vi "Winch_RT.vi"() -> ()   [LabVIEW 2018]
uses:
  Custom Controls/Address_Value Command Cluster.ctl
  Custom Controls/Counter.ctl
  Custom Controls/Slave_ID.ctl
  Custom Controls/MotorStatusCluster.ctl
  <vilib>/Platform/TimedLoop/XDataNode/timing_clust.ctl
  <vilib>/Platform/TimedLoop/XDataNode/nitl_modes.ctl
  <vilib>/Platform/TimedLoop/XDataNode/wakeup.ctl
  <vilib>/myRIO/Common/Instrument Driver Framework/myRIO v1.0/Encoder/typedefs/Encoder Signal Mode.ctl
  <vilib>/myRIO/Instrument Drivers/Onboard IO/Encoder/typedefs/Encoder Reference.ctl
  <vilib>/myRIO/Common/Instrument Driver Framework/Utilities/typedefs/myRIO Generic Hardware Reference.ctl
  <vilib>/myRIO/Common/Instrument Driver Framework/Utilities/typedefs/Hardware Version Enum.ctl
  <vilib>/myRIO/Common/Instrument Driver Framework/Utilities/typedefs/myRIO v1.0 Reference.ctl
  <vilib>/myRIO/Common/Instrument Driver Framework/Utilities/typedefs/Generic FPGA Reference.ctl
  <vilib>/myRIO/Common/Instrument Driver Framework/myRIO v1.0/Encoder/typedefs/Encoder Channels Enum.ctl
  <vilib>/myRIO/Common/Instrument Driver Framework/myRIO v1.0/Encoder/typedefs/Encoder Configuration v1.0.ctl
  <vilib>/userdefined/High Color/nirio_resource_hc.ctl
  <vilib>/myRIO/Instrument Drivers/Onboard IO/DIO/typedefs/DIO Reference.ctl
  <vilib>/myRIO/Common/Instrument Driver Framework/myRIO v1.0/DIO/typedefs/DIO Channels List.ctl
  <vilib>/myRIO/Common/Instrument Driver Framework/myRIO v1.0/DIO/typedefs/DIO Channels Enum.ctl
  <vilib>/myRIO/Common/Instrument Driver Framework/Utilities/vis/Is FPGA Ref Available.vi
  <vilib>/myRIO/Common/Instrument Driver Framework/myRIO v1.0/Encoder/vis/myRIO v1.1 Open Encoder.vi
  <vilib>/myRIO/Instrument Drivers/Onboard IO/Encoder/vis/Read.vi
  <vilib>/myRIO/Common/Instrument Driver Framework/myRIO v1.0/DIO/vis/myRIO v1.1 Open DIO.vi
  <vilib>/myRIO/Instrument Drivers/Onboard IO/DIO/vis/Read.vi
  <vilib>/myRIO/Common/Instrument Driver Framework/Utilities/vis/Validate Channels.vi
  <vilib>/myRIO/Common/Instrument Driver Framework/myRIO v1.0/Encoder/vis/myRIO v1.0 Reserve Encoder.vi
  <vilib>/myRIO/Common/Instrument Driver Framework/myRIO v1.0/DIO/vis/myRIO v1.0 Reserve DIO.vi
  <vilib>/myRIO/Common/Instrument Driver Framework/myRIO v1.0/UART/vis/myRIO v1.0 Close UART.vi
  <vilib>/myRIO/Common/Instrument Driver Framework/myRIO v1.0/Encoder/vis/myRIO v1.0 Build MUX Configuration Encoder.vi
  <vilib>/myRIO/Common/Instrument Driver Framework/myRIO v1.0/Resource Manager/vis/myRIO v1.0 Reserve Channel List.vi
  <vilib>/myRIO/Common/Instrument Driver Framework/myRIO v1.0/DIO/vis/myRIO v1.0 Build MUX Configuration DIO.vi
  <vilib>/myRIO/Common/Instrument Driver Framework/myRIO v1.0/Resource Manager/vis/myRIO v1.0 Create Configuration List.vi
  <vilib>/myRIO/Common/Instrument Driver Framework/myRIO v1.0/Resource Manager/vis/myRIO v1.0 Reserve Channel.vi
  <vilib>/myRIO/Common/Instrument Driver Framework/myRIO v1.0/Resource Manager/vis/myRIO v1.0 Unreserve Channel.vi
  <vilib>/myRIO/Common/Instrument Driver Framework/myRIO v1.0/Resource Manager/vis/myRIO v1.0 Build Mutex Name.vi
  <vilib>/Plasmionique/MB Master/MB_Master_Serial/MB_Master_Serial.lvclass
  D:/Program Files (x86)/National Instruments/LabVIEW 2018/vi.lib/Plasmionique/MB Master/MB_Master/MB_Master.lvclass
  <vilib>/Utility/VariantDataType/GetNumericInfo.vi
  <vilib>/Utility/error.llb/Error Cluster From Error Code.vi
  <vilib>/myRIO/Common/Instrument Driver Framework/myRIO v1.0/myRIO v1.1 Open.vi
  <vilib>/myRIO/Common/Instrument Driver Framework/Utilities/vis/IO Manager.vi
  <vilib>/myRIO/Common/Instrument Driver Framework/Utilities/vis/Configuration Manager.vi
  <vilib>/myRIO/Common/Instrument Driver Framework/myRIO v1.0/Resource Manager/vis/myRIO v1.0 Configure IO.vi
  <vilib>/myRIO/Common/Instrument Driver Framework/myRIO v1.0/myRIO v1.0 Close.vi
  <vilib>/myRIO/Common/Instrument Driver Framework/myRIO v1.0/Encoder/vis/myRIO v1.0 Configure Encoder.vi
  <vilib>/myRIO/Common/Instrument Driver Framework/myRIO v1.0/Encoder/vis/myRIO v1.0 Read Encoder.vi
  <vilib>/myRIO/Common/Instrument Driver Framework/myRIO v1.0/DIO/vis/myRIO v1.0 Read DIO.vi
  <vilib>/myRIO/Common/Instrument Driver Framework/Utilities/vis/FPGA Ref Manager.vi
  <vilib>/myRIO/Common/Instrument Driver Framework/myRIO v1.0/myRIO v1.0 Reset FPGA.vi
  <vilib>/myRIO/Common/Instrument Driver Framework/myRIO v1.0/IRQ/vis/myRIO v1.0 IRQ Info FGV.vi
  <vilib>/myRIO/Common/Instrument Driver Framework/myRIO v1.0/IRQ/vis/myRIO v1.0 Timer IRQ Info FGV.vi
  <vilib>/myRIO/Common/Instrument Driver Framework/myRIO v1.0/IRQ/vis/myRIO v1.0 ISR Agent.vi
  <vilib>/platform/TimedLoop/XDataNode/XDataNode.xnode
  <vilib>/myRIO/Express VI/Onboard IO/Encoder/Encoder Express VI.xnode
  <vilib>/myRIO/Instrument Drivers/Onboard IO/Encoder/vis/myRIO Encoder Open.xnode
  <vilib>/myRIO/Express VI/Onboard IO/DI/DI Express VI.xnode
  <vilib>/myRIO/Instrument Drivers/Onboard IO/DIO/vis/myRIO DIO Open.xnode
  <vilib>/Plasmionique/MB Master/MB Master.lvlib
  <vilib>/Platform/TimedLoop/XDataNode/XDNodeRunTimeDep.lvlib
  <vilib>/myRIO/Instrument Drivers/Onboard IO/DIO/DIO.lvlib
  <vilib>/myRIO/Instrument Drivers/Utilities/Utilities.lvlib
  <vilib>/myRIO/Instrument Drivers/Onboard IO/Encoder/Encoder.lvlib
panel:
  in  "Tab Control":enum32{"Home", "Configuration"}(tab)
  out "error out (myRIO I/O)":errorcluster
  in  "Command to send (E3)":T1(radio)=enum."STOP"
  in  "Command to send (P2)":T2(radio)=enum."STOP"
  out "error out (MODBUS)":errorcluster
  out "Counter (P2)":T3
  in  "Reset Counter (P2)":bool caption="Reset"
  out "Overflow? (P2)":bool caption="Overflow?"
  out "Counter (E3)":T3
  out "Overflow? (E3)":bool caption="Overflow?"
  in  "Reset Counter (E3)":bool caption="Reset"
  out "LEFT PROXIMITY SENSOR (C/DIO1)":bool caption="LEFT PROXIMITY SENSOR"
  out "RIGHT PROXIMITY SENSOR (C/DIO3)":bool caption="RIGHT PROXIMITY SENSOR"
  out "Registers (P2)":i16[](array[numeric])
  out "Command History (P2)":cluster{"Command":T4, "Timestamp":timestamp}[](array[cluster]) {"Command"."Reg Address" format="%04b"}
  out "Registers (E3)":i16[](array[numeric])
  out "Command History (E3)":cluster{"Command":T4, "Timestamp":timestamp}[](array[cluster]) {"Command"."Reg Address" format="%04b"}
  out "Motor Status (P2)":T5={"State"=0, "Direction"="TETHER IN", "Speed"=150} {"State" items=["OFF", "ON"]; "Speed" min=-1000 max=1000 step=1}
  out "Motor Status (E3)":T5={"State"=0, "Direction"="MOVE RIGHT", "Speed"=10} {"State" items=["OFF", "ON"]; "Speed" min=-1000 max=1000 step=1}
  in  "Mode (RTU)":enum16{"RTU", "ASCII"}(ring)
  in  "Serial Config":T6={"baud rate (bps)"=115200, "stop bits"=10, "parity"=0, "flow control"=0, "timeout"=3000, "retries"=5} {"stop bits" items=["1.0"=10, "1.5"=15, "2.0"=20]; "flow control" items=["None", "XON/XOFF", "RTS/CTS", "XON/XOFF & RTS/CTS", "DTR/DSR", "XON/XOFF & DTR/DSR"]; "parity" items=["None", "Odd", "Even", "Mark", "Space"]}
  in  "VISA Resource":refnum<visa-resource-name>="ASRL3::INSTR"
  in  "Configuration Tab Control":enum32{"P2 VFD", "E3 VFD"}(tab)
  in  "P2 Command List":T4[](array[typedef])=[{"Reg Address"=0, "Value"=1, "Dirrection"="START"}, {"Reg Address"=0, "Value"=0, "Dirrection"="STOP"}, {"Reg Address"=1, "Value"=150, "Dirrection"="TETHER IN"}, {"Reg Address"=1, "Value"=-150, "Dirrection"="TETHER OUT"}] {"Value" min=-1000 max=1000 step=1; "Reg Address" format="%04x"}
  out "Slave ID (P2)":T7=1 items=["P2 VFD"=1, "E3 VFD"=2]
  in  "E3 Command List":T4[](array[typedef])=[{"Reg Address"=0, "Value"=1, "Dirrection"="START"}, {"Reg Address"=0, "Value"=0, "Dirrection"="STOP"}, {"Reg Address"=1, "Value"=10, "Dirrection"="MOVE RIGHT"}, {"Reg Address"=1, "Value"=-10, "Dirrection"="MOVE LEFT"}] {"Value" min=-1000 max=1000 step=1; "Reg Address" format="%04x"}
  out "Slave ID (E3)":T7=2 items=["P2 VFD"=1, "E3 VFD"=2]
  in  "Period (myRIO I/O Loop)":i64=100
  in  "Period (MODBUS Loop)":i64=100
  in  "stop":bool
  # "WINCH CONTROL SYSTEM"
  # "P2 VFD"
  # "E3 VFD"
  # "Communication Parameters"
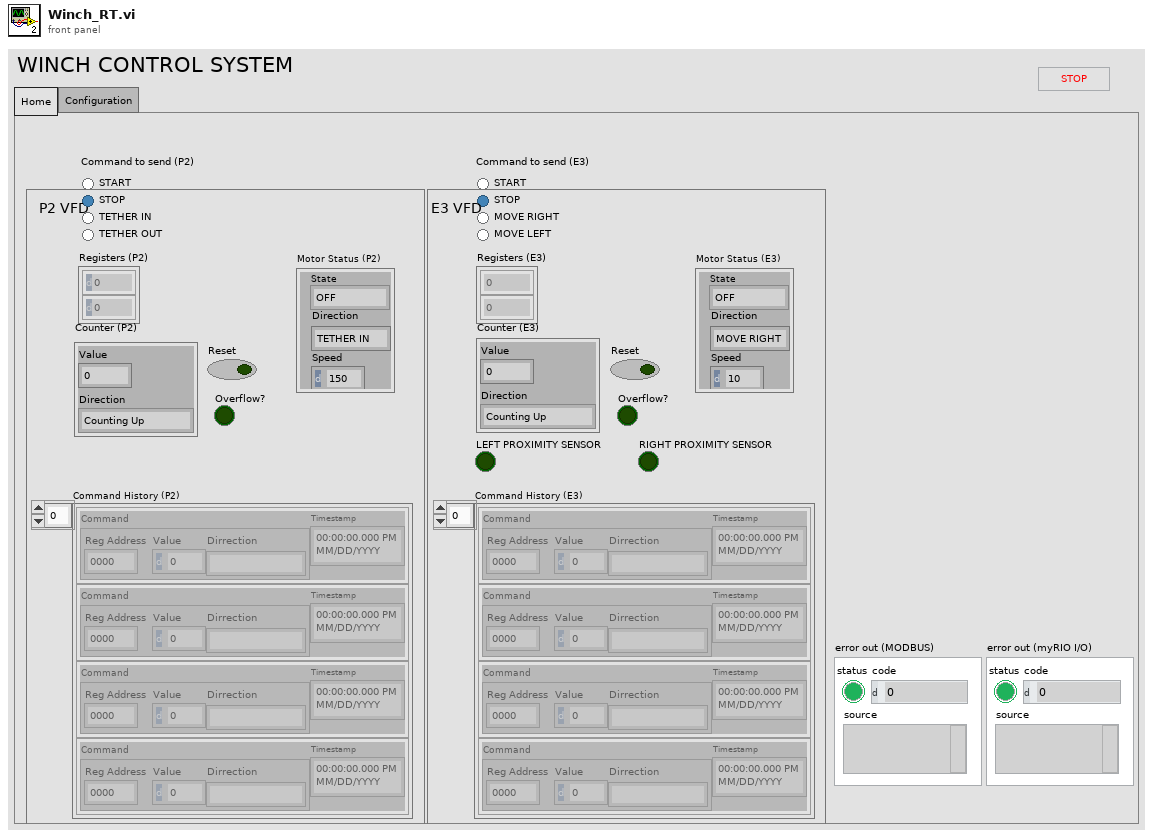
[diagram p1: front panel]
types:
  T1 = enum32{"START", "STOP", "MOVE RIGHT", "MOVE LEFT"}
  T2 = enum32{"START", "STOP", "TETHER IN", "TETHER OUT"}
  T3 = typedef "Counter.ctl" = cluster{"Value":i32, "Direction":enum16{"Counting Up", "Counting Down"}}
  T4 = typedef "Address_Value Command Cluster.ctl" = cluster{"Reg Address":u16, "Value":i16, "Dirrection":string}
  T5 = typedef "MotorStatusCluster.ctl" = cluster{"State":i16, "Direction":string, "Speed":i16}
  T6 = cluster{"baud rate (bps)":u32, "stop bits":u16, "parity":u16, "flow control":u16, "timeout":u32, "retries":i32}
  T7 = typedef "Slave_ID.ctl" = u8
  T8 = typedef "XDNodeRunTimeDep.lvlib/timing_clust.ctl" = cluster{"Expected End [f-1]":u64, "Actual End [f-1]":u64, "Finished Late? [f-1]":bool, "Expected End [i-1]":u64, "Actual End [i-1]":u64, "Finished Late? [i-1]":bool, "Expected Start [i]":u64, "Actual Start [i]":u64, "Expected Start [f]":u64, "Actual Start [f]":u64, "Source Name":string, "Structure Name":string, "Period":i64, "Deadline":i64, "Offset":i64, "Start":i64, "Priority":i32, "Timeout":i32, "Mode":T9, "Wakeup Reason":T10, "Error":errorcluster, "Source Type":string, "Secondary Source Type":string, "Global End Time":u64, "Global Start Time":u64, "Frame Duration":u64, "Iteration Duration":u64, "Assigned CPU":i32, "I/O Scan Engine Mode":u32}
  T9 = typedef "XDNodeRunTimeDep.lvlib/nitl_modes.ctl" = enum32{"No Change", "Process missed periods, maintain original phase", "Discard missed periods, maintain original phase", "Process missed periods, ignore original phase", "Discard missed periods, ignore original phase"}
  T10 = typedef "XDNodeRunTimeDep.lvlib/wakeup.ctl" = enum32{"Normal", "Aborted", "Asynchronous wakeup", "Timing source error", "Timed loop error", "Timeout"}
  T11 = cluster{"Register/Value Command Cluster":T4, "seconds since 1Jan1904":timestamp}
  T12 = typedef "Encoder.lvlib/Encoder Reference.ctl" = cluster{"myRIO Reference":T13, "Encoder Channels Enum":T17}
  T13 = typedef "myRIO Generic Hardware Reference.ctl" = cluster{"myRIO Model":T14, "myRIO Hardware Reference":T15}
  T14 = typedef "Hardware Version Enum.ctl" = enum16{"Unknown", "myRIO-1900", "myRIO-1950", "roboRIO", "NI ELVIS RIO CM", "ELVIS III"}
  T15 = typedef "myRIO v1.0 Reference.ctl" = cluster{"Generic FPGA Reference":T16, "Allow multiple opens":bool}
  T16 = typedef "Generic FPGA Reference.ctl" = refnum<k20>
  T17 = typedef "Encoder Channels Enum.ctl" = enum16{"Not Connected", "C/ENC0", "C/ENC1", "A/ENC", "A/ENC0", "A/ENC1", "A/ENC2", "A/ENC3", "A/ENC4", "A/ENC5", "A/ENC6", "A/ENC7", "A/ENC8", "A/ENC9", "B/ENC", "B/ENC0", "B/ENC1", "B/ENC2", "B/ENC3", "B/ENC4", "B/ENC5", "B/ENC6", "B/ENC7", "B/ENC8", "B/ENC9", "DIO/ENC0", "DIO/ENC1", "DIO/ENC2", "DIO/ENC3", "DIO/ENC4"}
  T18 = typedef "Encoder Signal Mode.ctl" = enum16{"Quadrature phase signal", "Step and direction signal"}
  T19 = typedef "nirio_resource_hc.ctl" = tag
  T20 = typedef "DIO.lvlib/DIO Reference.ctl" = cluster{"myRIO Reference":T13, "DIO Channels List":T21}
  T21 = typedef "DIO Channels List.ctl" = T22[]
  T22 = typedef "DIO Channels Enum.ctl" = enum16{"Not Connected", "C/DIO0", "C/DIO1", "C/DIO2", "C/DIO3", "C/DIO4", "C/DIO5", "C/DIO6", "C/DIO7", "A/DIO0", "A/DIO1", "A/DIO2", "A/DIO3", "A/DIO4", "A/DIO5", "A/DIO6", "A/DIO7", "A/DIO8", "A/DIO9", "A/DIO10", "A/DIO11", "A/DIO12", "A/DIO13", "A/DIO14", "A/DIO15", "A/DIO16", "A/DIO17", "A/DIO18", "A/DIO19", "B/DIO0", "B/DIO1", "B/DIO2", "B/DIO3", "B/DIO4", "B/DIO5", "B/DIO6", "B/DIO7", "B/DIO8", "B/DIO9", "B/DIO10", "B/DIO11", "B/DIO12", "B/DIO13", "B/DIO14", "B/DIO15", "B/DIO16", "B/DIO17", "B/DIO18", "B/DIO19", "LED0", "LED1", "LED2", "LED3", "Button0", "DIO/DIO0", "DIO/DIO1", "DIO/DIO2", "DIO/DIO3", "DIO/DIO4", "DIO/DIO5", "DIO/DIO6", "DIO/DIO7", "DIO/DIO8", "DIO/DIO9", "SPI/CS0", "SPI/CS1", "SPI/CS2", "SPI/CS3", "LED RADIO (Green)", "LED RADIO (Red)", "LED COMM (Green)", "LED COMM (Red)", "LED MODE (Green)", "LED MODE (Red)"}
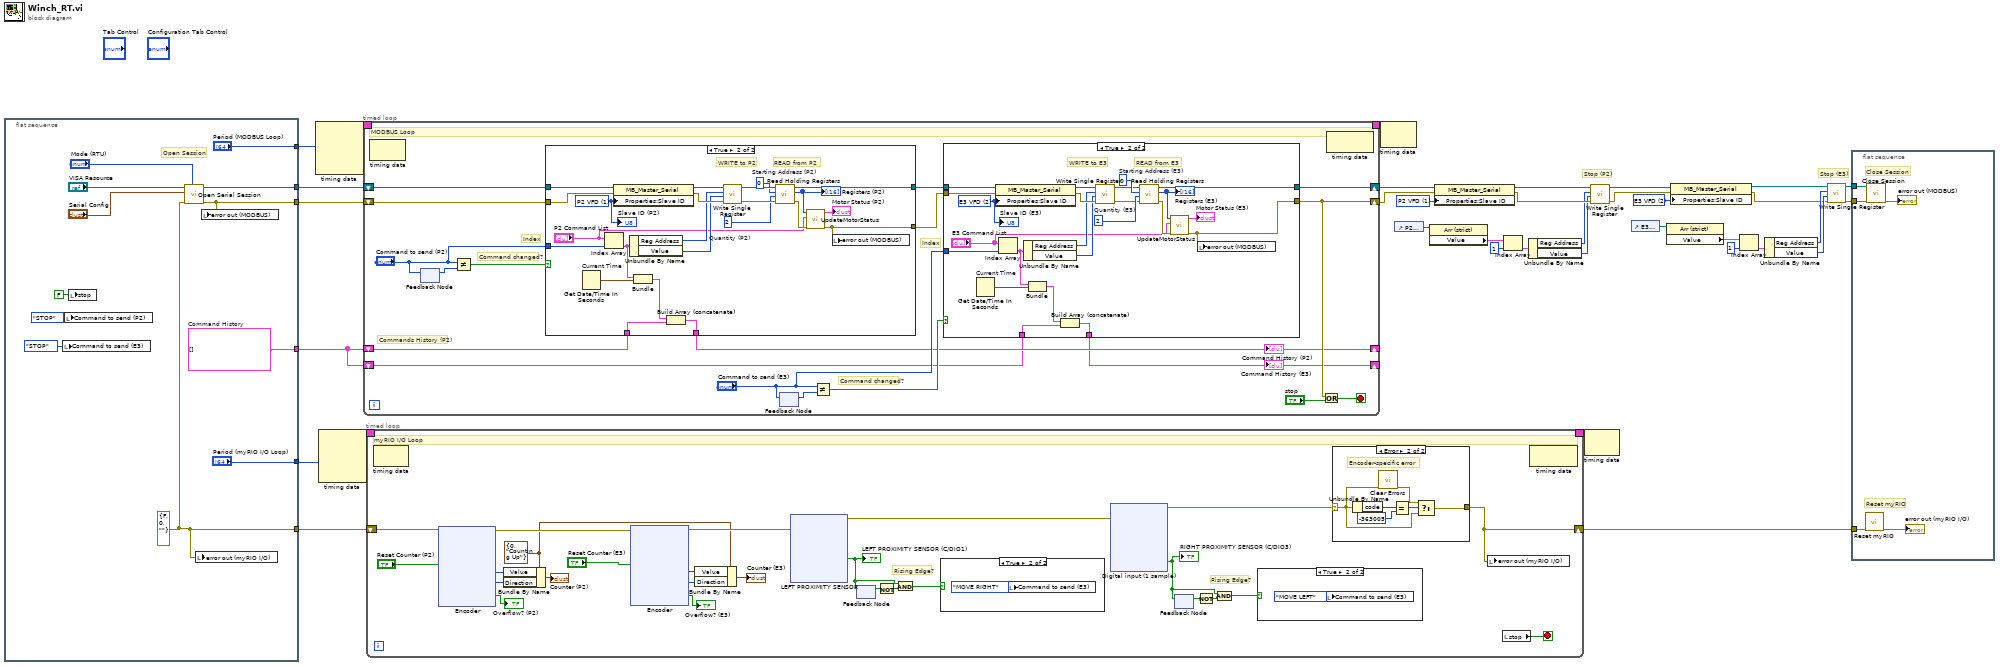
[diagram p0: block diagram]
diagram:
  w5 = T7 2 items=["P2 VFD"=1, "E3 VFD"=2] ("Slave ID")
  w24 = T7 1 items=["P2 VFD"=1, "E3 VFD"=2] ("Slave ID")
  # "Stop (E3)"
  # "Stop (P2)"
  n1 = flat-sequence {
    tunnel: [w44] -> w35
    tunnel: [w42] -> w34
    tunnel: ["Period (myRIO I/O Loop)"] -> w31
    tunnel: [w37] -> w30
    tunnel: [w38] -> w25
    tunnel: ["Period (MODBUS Loop)"] -> w26
    frame #0 {
      w38 = cluster{"Command":T4, "Timestamp":timestamp}[] []  # Command History
      w37 = errorcluster {"status"=FALSE, "code"=0, "source"=""} ("error out (myRIO I/O)")
      # "Open Session"
      n2 = local write "Command to send (E3)"(T1."STOP" ("Command to send (E3)")) -> ()
      n3 = local write "Command to send (P2)"(T2."STOP" ("Command to send (P2)")) -> ()
      n4 = local write "stop"(FALSE ("stop")) -> ()
      n5 = call <vilib>:"Open Serial Session.vi"("Mode (RTU)"="Mode (RTU)", "Error in"=w37, "Serial Config"="Serial Config", "VISA Resource"="VISA Resource") -> ("Error out"=w42:errorcluster, "MB_Serial session"=w44:refnum<class "MB_Master_Serial.lvclass">)  [unwired: 6 in]
      n6 = local write "error out (myRIO I/O)"(w37) -> ()
      n7 = local write "error out (MODBUS)"(w42) -> ()
    }
  }
  n8 = node-c288(w26) -> (w28:T8)  [unwired: 3 in]
  n9 = node-c288(w31) -> (w33:T8)  [unwired: 3 in]
  n10 = timed-loop {
    shift-right: [w61] -> w23
    shift-left: w35 -> [w65]
    shift-right: [w59] -> w22
    shift-left: w34 -> [w64]
    shift-right: [w50] -> _
    shift-left: w25 -> [w51]
    timing: w28 -> [_]
    timing-out: [_] -> w27
    shift-right: [w48] -> _
    shift-left: w25 -> [w49]
    stop <- w58 stop-if-true
    # "Commands History (P2)"
    # "Index"
    # "Index"
    # "Command changed?"
    # "Command changed?"
    # "MODBUS Loop"
    n11 = node-c288() -> ()  [unwired: 1 in, 1 out]
    n12 = feedback-in #1("Command to send (P2)") -> ()
    n13 = feedback #1() -> (w57:T2)  [unwired: 1 in]
    n14 = Not Equal?(x="Command to send (P2)", y=w57) -> (x != y?=w56:bool)
    n15 = case shown="True" w56 {
      tunnel: w65 -> [w96 w119]
      tunnel: w64 -> [w95 w118]
      tunnel: [w96 w117] -> w63
      tunnel: [w95 w98] -> w62
      tunnel: "Command to send (P2)" -> [_ w108]
      tunnel: w51 -> [w94 w104]
      tunnel: [w94 w103] -> w50
      frame False {
      }
      frame True {
        w114 = u16 2  # Quantity (P2)
        w110 = T7 1 items=["P2 VFD"=1, "E3 VFD"=2] ("Slave ID")
        w113 = u16 0  # Starting Address (P2)
        # "READ from P2"
        # "WRITE to P2"
        n16 = Get Date/Time In Seconds "Current Time"() -> (seconds since 1Jan1904=w106:timestamp)
        n17 = Index Array(array="P2 Command List", index=w108) -> (element=w107:T4)
        n18 = property class="MB_Master_Serial"(reference=w119, error in=w118, "Properties:Slave ID"=w110) -> (reference out=w112:refnum<class "MB_Master_Serial.lvclass">, error out=w111:errorcluster)
        n19 = Unbundle By Name(w107) -> ("Reg Address"=w109:u16, "Value"=w102:i16)
        n20 = Bundle("Register/Value Command Cluster"=w107, "seconds since 1Jan1904"=w106) -> (w105:T11)  [unwired: 1 in]
        n21 = Build Array (concatenate)(w105, w104) -> (w103:cluster{"Command":T4, "Timestamp":timestamp}[])
        n22 = call <vilib>:"Write Single Register.vi"("error in (no error)"=w111, "value"=w102, "address"=w109, "MB session in"=w112) -> ("error out"=w115:errorcluster, "MB session out"=w116:refnum<class "MB_Master_Serial.lvclass">)  [unwired: 6 in]
        n23 = call <vilib>:"Read Holding Registers.vi"("error in (no error)"=w115, "quantity"=w114, "starting address"=w113, "MB session in"=w116) -> ("error out"=w101:errorcluster, "Registers"=w100:u16[], "MB session out"=w117:refnum<class "MB_Master_Serial.lvclass">)  [unwired: 5 in]
        "Registers (P2)" <- w100
        n24 = call "UpdateMotorStatus.vi"("error in (MODBUS)"=w101, "Command List"="P2 Command List", "Registers"=w100) -> ("error out (MODBUS)"=w98:errorcluster, "Motor Status"=→"Motor Status (P2)":T5)  [unwired: 7 in]
        n25 = local write "error out (MODBUS)"(w98) -> ()
        "Slave ID (P2)" <- w110
      }
    }
    "Command History (P2)" <- w50
    n26 = feedback #2() -> (w55:T1)  [unwired: 1 in]
    n27 = feedback-in #2("Command to send (E3)") -> ()
    n28 = Not Equal?(x="Command to send (E3)", y=w55) -> (x != y?=w54:bool)
    n29 = case shown="True" w54 {
      tunnel: w63 -> [w70 w93]
      tunnel: w62 -> [w69 w92]
      tunnel: [w70 w91] -> w61
      tunnel: [w69 w71] -> w59
      tunnel: "Command to send (E3)" -> [_ w83]
      tunnel: w49 -> [w68 w79]
      tunnel: [w68 w78] -> w48
      frame False {
      }
      frame True {
        w89 = u16 2  # Quantity (E3)
        w84 = T7 2 items=["P2 VFD"=1, "E3 VFD"=2] ("Slave ID")
        w90 = u16 0  # Starting Address (E3)
        # "READ from E3"
        # "WRITE to E3"
        n30 = Get Date/Time In Seconds "Current Time"() -> (seconds since 1Jan1904=w82:timestamp)
        n31 = property class="MB_Master_Serial"(reference=w93, error in=w92, "Properties:Slave ID"=w84) -> (reference out=w86:refnum<class "MB_Master_Serial.lvclass">, error out=w85:errorcluster)
        n32 = Index Array(array="E3 Command List", index=w83) -> (element=w80:T4)
        n33 = Unbundle By Name(w80) -> ("Reg Address"=w77:u16, "Value"=w76:i16)
        n34 = Bundle("Register/Value Command Cluster"=w80, "seconds since 1Jan1904"=w82) -> (w81:T11)  [unwired: 1 in]
        n35 = Build Array (concatenate)(w81, w79) -> (w78:cluster{"Command":T4, "Timestamp":timestamp}[])
        n36 = call <vilib>:"Write Single Register.vi"("error in (no error)"=w85, "value"=w76, "address"=w77, "MB session in"=w86) -> ("error out"=w88:errorcluster, "MB session out"=w87:refnum<class "MB_Master_Serial.lvclass">)  [unwired: 6 in]
        n37 = call <vilib>:"Read Holding Registers.vi"("error in (no error)"=w88, "quantity"=w89, "starting address"=w90, "MB session in"=w87) -> ("error out"=w74:errorcluster, "Registers"=w73:u16[], "MB session out"=w91:refnum<class "MB_Master_Serial.lvclass">)  [unwired: 5 in]
        "Registers (E3)" <- w73
        n38 = call "UpdateMotorStatus.vi"("error in (MODBUS)"=w74, "Command List"="E3 Command List", "Registers"=w73) -> ("error out (MODBUS)"=w71:errorcluster, "Motor Status"=→"Motor Status (E3)":T5)  [unwired: 7 in]
        n39 = local write "error out (MODBUS)"(w71) -> ()
        "Slave ID (E3)" <- w84
      }
    }
    "Command History (E3)" <- w48
    n40 = Or(x=w59, y="stop") -> (x .or. y?=w58:bool)
    n41 = node-c288() -> ()  [unwired: 1 in, 1 out]
  }
  n42 = timed-loop {
    timing: w33 -> [_]
    timing-out: [_] -> w32
    shift-right: [w142] -> w29
    shift-left: w30 -> [w140]
    stop <- w144 stop-if-true
    w129 = T3 {"Value"=0, "Direction"=enum."Counting Up"} ("Counter")
    # "Rising Edge?"
    # "Rising Edge?"
    # "myRIO I/O Loop"
    n43 = node-c288() -> ()  [unwired: 1 in, 1 out]
    n44 = xnode "Encoder"("Reset Counter"="Reset Counter (P2)", "error in (no error)"=w140) -> ("Counter Value"=w130:i32, "Counter Direction"=w131:enum16{"Counting Up", "Counting Down"}, "Overflow?"=→"Overflow? (P2)":bool, "error out"=w135:errorcluster)
    n45 = Bundle By Name(cluster=w129, "Value"=w130, "Direction"=w131) -> (→"Counter (P2)":T3)
    n46 = xnode "Encoder"("Reset Counter"="Reset Counter (E3)", "error in (no error)"=w135) -> ("Counter Value"=w136:i32, "Counter Direction"=w137:enum16{"Counting Up", "Counting Down"}, "Overflow?"=→"Overflow? (E3)":bool, "error out"=w132:errorcluster)
    n47 = Bundle By Name(cluster=w129, "Value"=w136, "Direction"=w137) -> (→"Counter (E3)":T3)
    n48 = xnode "LEFT PROXIMITY SENSOR"("error in (no error)"=w132) -> ("C/DIO1 (DIO1)"=w125:bool, "error out"=w145:errorcluster)
    "LEFT PROXIMITY SENSOR (C/DIO1)" <- w125
    n49 = feedback #3() -> (w127:bool)  [unwired: 1 in]
    n50 = feedback-in #3(w125) -> ()
    n51 = Not(x=w127) -> (.not. x?=w126:bool)
    n52 = And(x=w125, y=w126) -> (x .and. y?=w124:bool)
    n53 = case shown="True" w124 {
      frame False {
      }
      frame True {
        n54 = local write "Command to send (E3)"(T1."MOVE RIGHT" ("Command to send (E3)")) -> ()
      }
    }
    n55 = xnode "Digital input (1 sample)"("error in (no error)"=w145) -> ("C/DIO3 (DIO3)"=w121:bool, "error out"=w143:errorcluster)
    "RIGHT PROXIMITY SENSOR (C/DIO3)" <- w121
    n56 = feedback #4() -> (w122:bool)  [unwired: 1 in]
    n57 = feedback-in #4(w121) -> ()
    n58 = Not(x=w122) -> (.not. x?=w123:bool)
    n59 = And(x=w121, y=w123) -> (x .and. y?=w120:bool)
    n60 = case shown="True" w120 {
      frame False {
      }
      frame True {
        n61 = local write "Command to send (E3)"(T1."MOVE LEFT" ("Command to send (E3)")) -> ()
      }
    }
    n62 = case shown="Error" w143 {
      selector: w143 -> [w240 w242]
      tunnel: [w240 w241] -> w142
      frame No Error {
      }
      frame Error {
        # "Encoder-specific error"
        n63 = Unbundle By Name(w242) -> ("code"=w246:i32)
        n64 = call <vilib>:"Clear Errors.vi"("error in (no error)"=w242) -> ("error out"=w243:errorcluster)  [unwired: 5 in, 1 out]
        n65 = Equal?(x=w246, y=-363005) -> (x = y?=w244:bool)
        n66 = Select(t=w243, s=w244, f=w242) -> (s? t:f=w241:errorcluster)
      }
    }
    n67 = local write "error out (myRIO I/O)"(w142) -> ()
    n68 = local read "stop"() -> (w144:bool)
    n69 = node-c288() -> ()  [unwired: 1 in, 1 out]
  }
  n70 = node-c288(w27) -> ()  [unwired: 1 out]
  n71 = control-ref of="P2 Command List"() -> (w20:refnum<vi>)
  n72 = property class="Arr (strict)"(reference=w20) -> ("Value"=w19:T4[])  [unwired: 1 in, 2 out]
  n73 = property class="MB_Master_Serial"(reference=w23, error in=w22, "Properties:Slave ID"=w24) -> (reference out=w17:refnum<class "MB_Master_Serial.lvclass">, error out=w16:errorcluster)
  n74 = Index Array(array=w19, index=1) -> (element=w21:T4)
  n75 = Unbundle By Name(w21) -> ("Reg Address"=w15:u16, "Value"=w14:i16)
  n76 = node-c288(w32) -> ()  [unwired: 1 out]
  n77 = call <vilib>:"Write Single Register.vi"("error in (no error)"=w16, "value"=w14, "address"=w15, "MB session in"=w17) -> ("error out"=w3:errorcluster, "MB session out"=w4:refnum<class "MB_Master_Serial.lvclass">)  [unwired: 6 in]
  n78 = control-ref of="E3 Command List"() -> (w7:refnum<vi>)
  n79 = property class="Arr (strict)"(reference=w7) -> ("Value"=w8:T4[])  [unwired: 1 in, 2 out]
  n80 = property class="MB_Master_Serial"(reference=w4, error in=w3, "Properties:Slave ID"=w5) -> (reference out=w10:refnum<class "MB_Master_Serial.lvclass">, error out=w11:errorcluster)
  n81 = Index Array(array=w8, index=1) -> (element=w6:T4)
  n82 = Unbundle By Name(w6) -> ("Reg Address"=w12:u16, "Value"=w13:i16)
  n83 = call <vilib>:"Write Single Register.vi"("error in (no error)"=w11, "value"=w13, "address"=w12, "MB session in"=w10) -> ("error out"=w1:errorcluster, "MB session out"=w2:refnum<class "MB_Master_Serial.lvclass">)  [unwired: 6 in]
  n84 = flat-sequence {
    tunnel: w29 -> [w322]
    tunnel: w2 -> [w320]
    tunnel: w1 -> [w319]
    frame #0 {
      # "Reset myRIO"
      # "Close Session"
      n85 = call <vilib>:"Reset myRIO.vi"("error in (no error)"=w322) -> ("error out"=→"error out (myRIO I/O)":errorcluster)  [unwired: 10 in]
      n86 = call-dynamic "Close Session.vi"("error in (no error)"=w319, "MB_Serial session"=w320) -> ("error out"=→"error out (MODBUS)":errorcluster)  [unwired: 9 in]
    }
  }
